vi "Script Cases.vi"(0 "Primitives & Arguments":T1) -> ()   [LabVIEW 2014]
uses:
  Begin/Global Variables.vi
  Begin/Global RefNums.vi
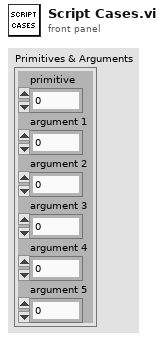
[diagram p1: front panel]
types:
  T1 = cluster{"primitive":i32, "argument 1":dbl, "argument 2":dbl, "argument 3":dbl, "argument 4":dbl, "argument 5":dbl}
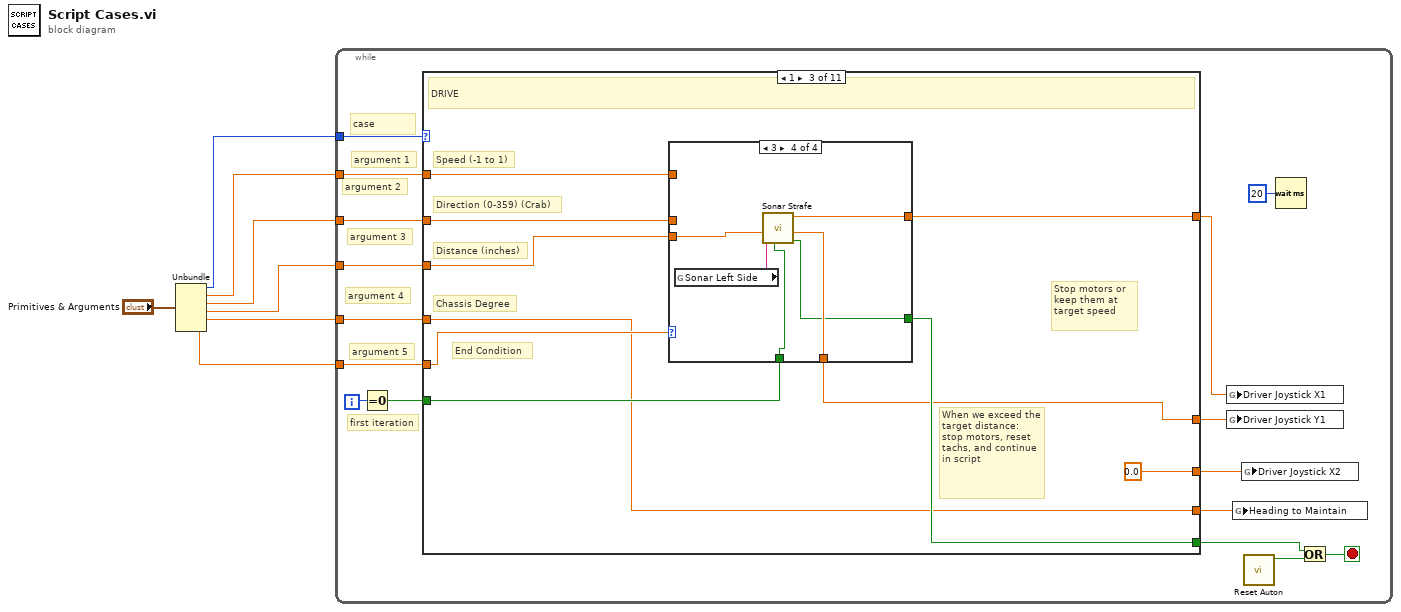
[diagram p0: block diagram]
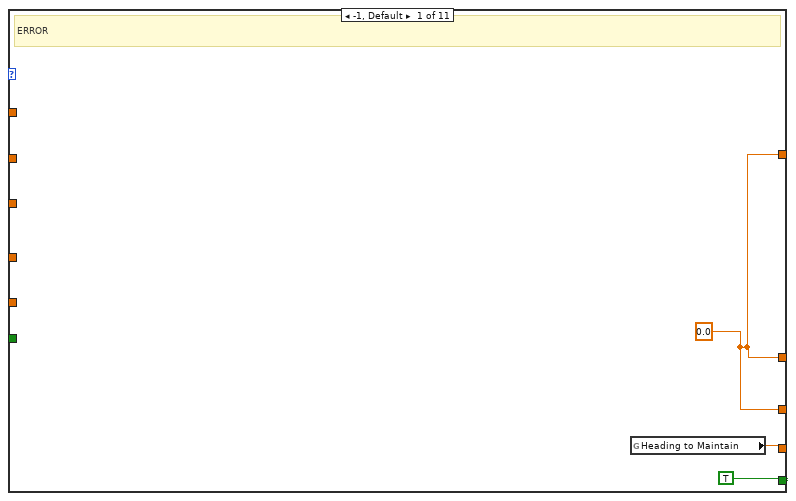
[diagram p2: hidden frame]
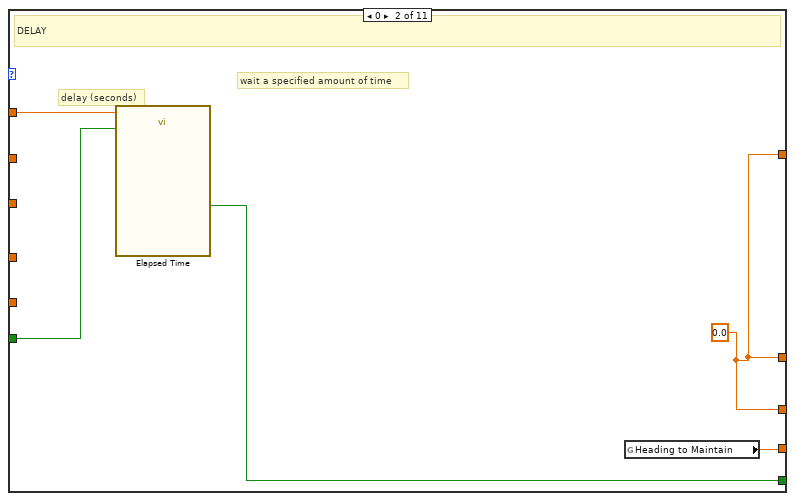
[diagram p3: hidden frame]
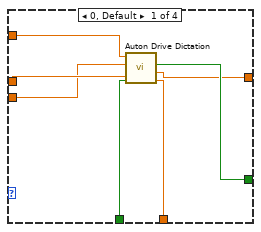
[diagram p4: hidden frame]
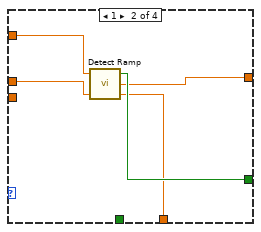
[diagram p5: hidden frame]
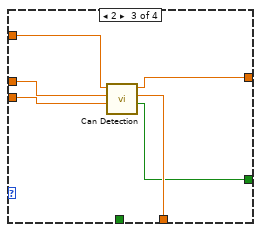
[diagram p6: hidden frame]
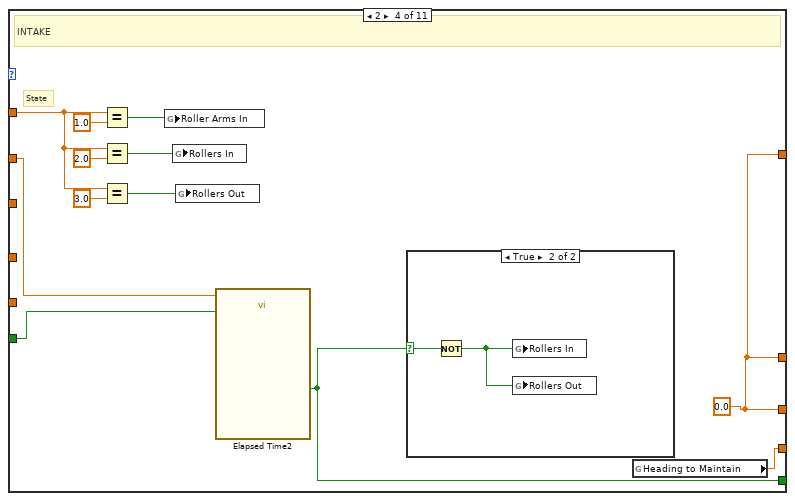
[diagram p7: hidden frame]
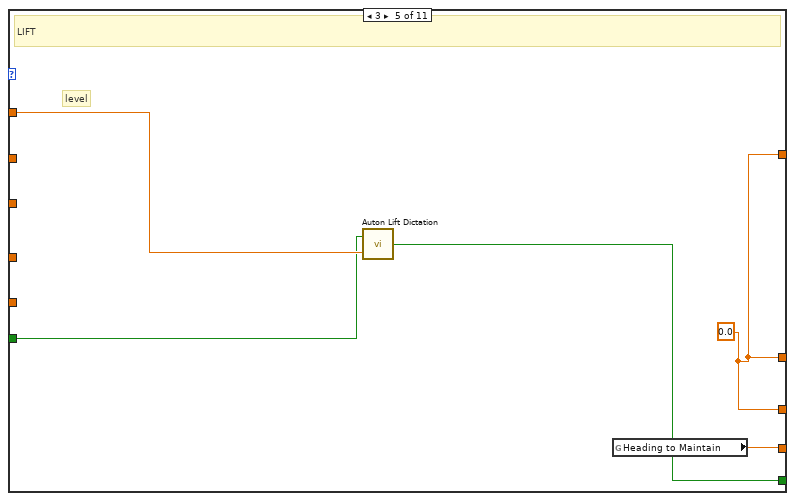
[diagram p9: hidden frame]
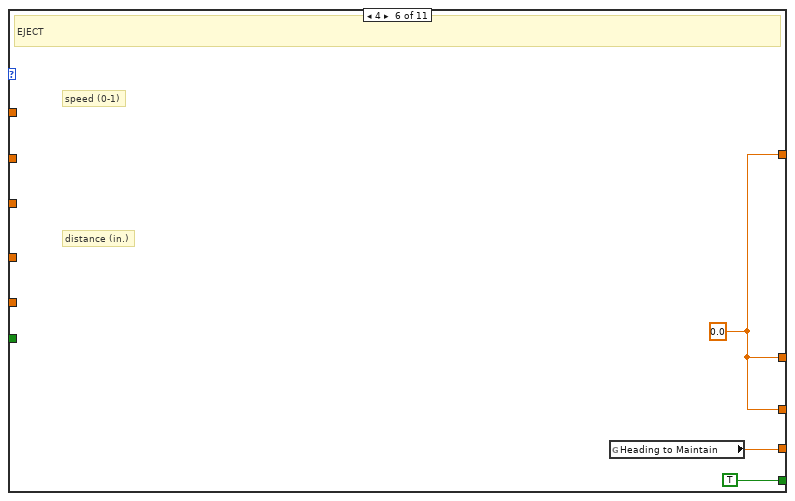
[diagram p10: hidden frame]
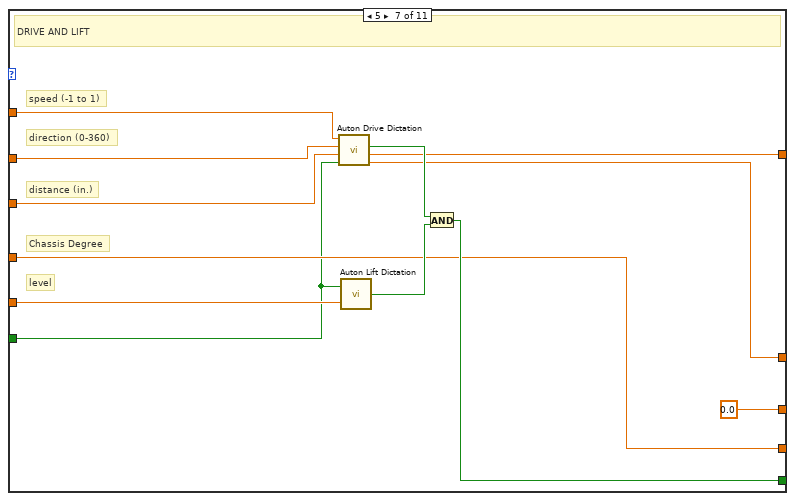
[diagram p11: hidden frame]
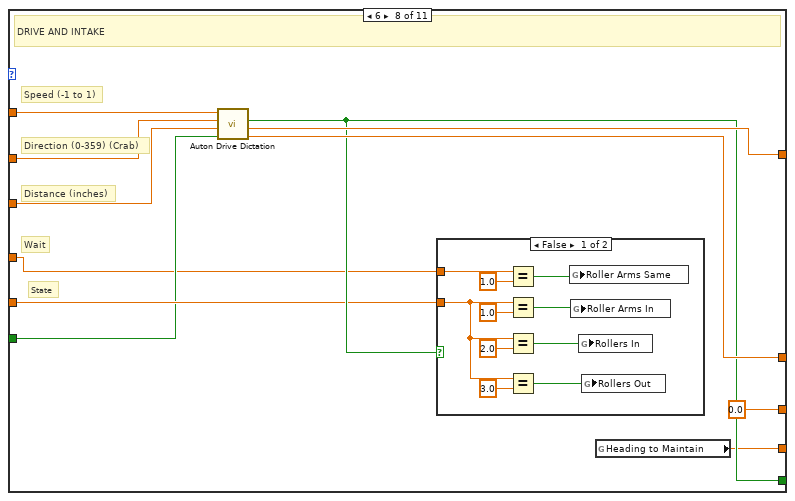
[diagram p12: hidden frame]
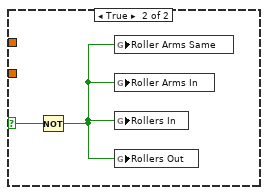
[diagram p13: hidden frame]
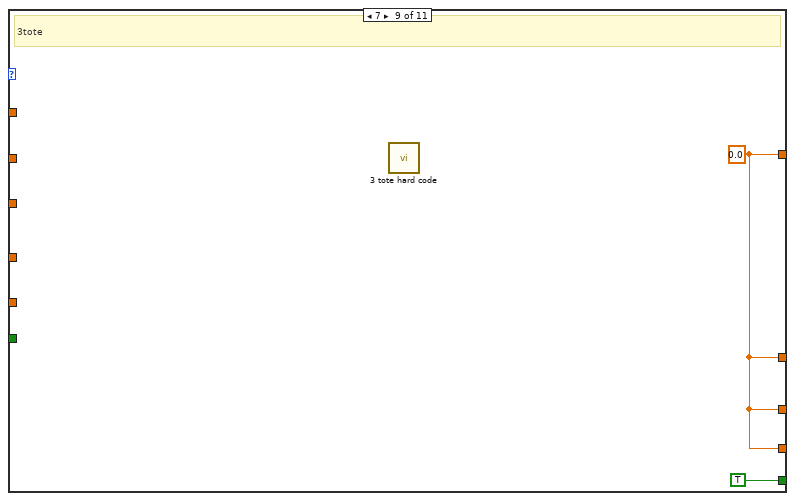
[diagram p14: hidden frame]
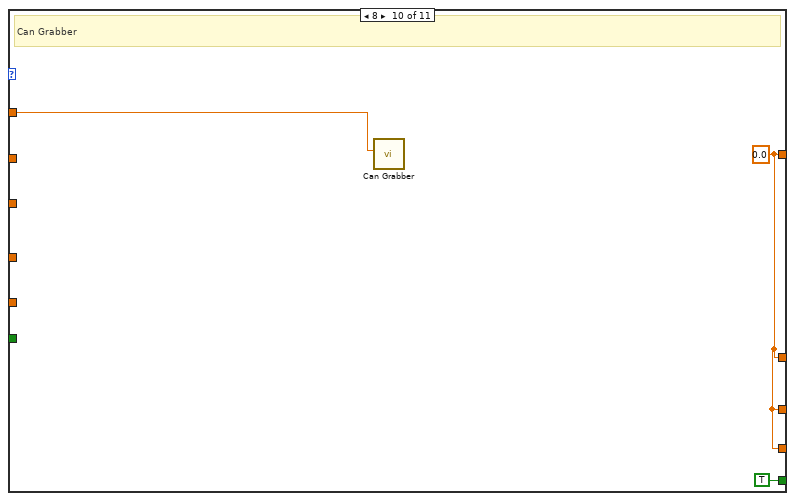
[diagram p15: hidden frame]
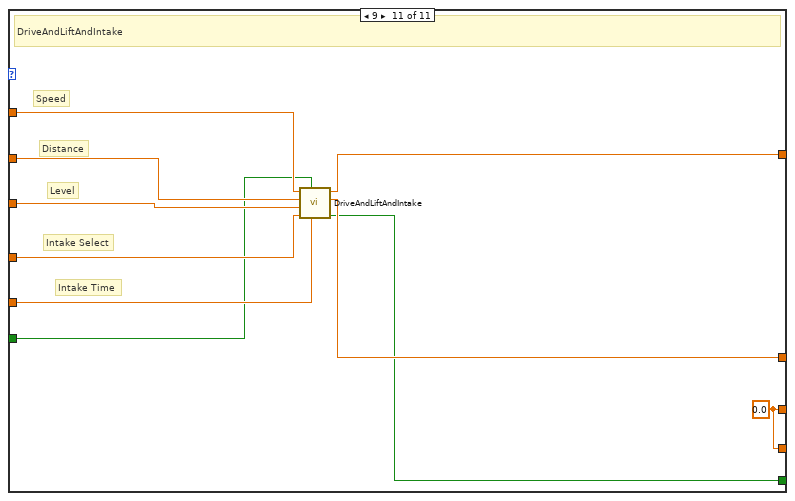
[diagram p16: hidden frame]
diagram:
  n1 = Unbundle("Primitives & Arguments") -> ("primitive"=w6:i32, "argument 1"=w5:dbl, "argument 2"=w4:dbl, "argument 3"=w3:dbl, "argument 4"=w2:dbl, "argument 5"=w1:dbl)
  n2 = while {
    tunnel: w5 -> [w23]
    tunnel: w4 -> [w22]
    tunnel: w3 -> [w21]
    tunnel: w2 -> [w20]
    tunnel: w1 -> [w19]
    tunnel: w6 -> [w18]
    i -> [w17]
    stop <- w9 stop-if-true
    # "first iteration"
    # "case"
    # "argument 5"
    # "argument 4"
    # "argument 3"
    # "argument 2"
    # "argument 1"
    n3 = Equal To 0?(x=w17) -> (x = 0?=w16:bool)
    n4 = case shown="1" w18 {
      tunnel: w23 -> [_ w31 w40 w74 w84 _ w98 w110 _ w125 w137]
      tunnel: w22 -> [_ _ w39 w70 _ _ w97 w109 _ _ w136]
      tunnel: w21 -> [_ _ w38 _ _ _ w96 w108 _ _ w135]
      tunnel: w20 -> [_ _ w34 _ _ _ w89 w101 _ _ w133]
      tunnel: w19 -> [_ _ w35 _ _ _ w95 w103 _ _ w134]
      tunnel: [TRUE w29 w37 w69 w83 TRUE w92 w105 TRUE ("Distance Reached?") TRUE ("Distance Reached?") w130] -> w10
      tunnel: w16 -> [_ w30 w36 w68 w81 _ w88 w102 _ _ w128]
      tunnel: [w25 w28 0.0 ("argument 1") w67 w82 w86 0.0 ("argument 1") 0.0 ("argument 1") w123 w127 w129] -> w15
      tunnel: [w24 w27 w34 w66 w80 w85 w89 w100 w123 w127 w129] -> w14
      tunnel: [w25 w28 w33 w67 w82 w86 w91 w107 w123 w127 w132] -> w12
      tunnel: [w25 w28 w32 w67 w82 w86 w90 w106 w123 w127 w131] -> w11
      frame -1, Default {
        w25 = 0.0 ("argument 1")
        # "ERROR"
        n5 = global read "Global Variables.vi" "Heading to Maintain"() -> (w24:dbl)
      }
      frame 0 {
        w28 = 0.0 ("argument 1")
        # "wait a specified amount of time"
        # "delay (seconds)"
        # "DELAY"
        n6 = call "Elapsed Time"("Time Target (s)"=w31, "Reset"=w30) -> ("Time has Elapsed"=w29:bool)  [unwired: 10 in, 7 out]
        n7 = global read "Global Variables.vi" "Heading to Maintain"() -> (w27:dbl)
      }
      frame 1 {
        # "Chassis Degree"
        # "End Condition"
        # "When we exceed the target distance: stop motors, reset tachs, and continue in script"
        # "Stop motors or keep them at target speed"
        # "Distance (inches)"
        # "Direction (0-359) (Crab)"
        # "Speed (-1 to 1)"
        # "DRIVE"
        n8 = case shown="3" w35 {
          tunnel: w40 -> [w48 w53 w57 _]
          tunnel: w39 -> [w47 w52 w56 _]
          tunnel: w38 -> [w46 _ w55 w65]
          tunnel: [w45 w51 w54 w62] -> w37
          tunnel: w36 -> [w44 _ _ w60]
          tunnel: [w43 w50 w59 w64] -> w33
          tunnel: [w42 w49 w58 w63] -> w32
          frame 0, Default {
            n9 = call "Auton Drive Dictation.vi"("Reset Encoders"=w44, "Distance (inches)"=w46, "Direction (0-359)"=w47, "Speed (-1 to 1)"=w48) -> ("Joy Y"=w42:dbl, "Joy X"=w43:dbl, "Distance Reached?"=w45:bool)  [unwired: 5 in]
          }
          frame 1 {
            n10 = call "Detect Ramp.vi"("Direction"=w52, "Speed"=w53) -> ("JoyY"=w49:dbl, "Joy X"=w50:dbl, "Finished"=w51:bool)  [unwired: 1 in]
          }
          frame 2 {
            n11 = call "Can Detection.vi"("Stop Voltage"=w55, "Direction (0-359)"=w56, "Speed"=w57) -> ("Distance Reached?"=w54:bool, "Joy Y"=w58:dbl, "Joy X"=w59:dbl)  [unwired: 6 in]
          }
          frame 3 {
            n12 = global read "Global RefNums.vi" "Sonar Left Side"() -> (w61:string)
            n13 = call "Sonar Strafe.vi"("reinitialize? (F)"=w60, "Sonar Side"=w61, "Desired Wall Distance"=w65) -> ("Distance Reached?"=w62:bool, "Joy Y"=w63:dbl, "Joy X"=w64:dbl)  [unwired: 6 in]
          }
        }
      }
      frame 2 {
        w67 = 0.0 ("argument 1")
        # "State"
        # "INTAKE"
        n14 = Equal?(x=w74, y=1.0) -> (x = y?=w71:bool)
        n15 = Equal?(x=w74, y=2.0) -> (x = y?=w72:bool)
        n16 = Equal?(x=w74, y=3.0) -> (x = y?=w73:bool)
        n17 = global write "Global Variables.vi" "Roller Arms In"(w71) -> ()
        n18 = global write "Global Variables.vi" "Rollers In"(w72) -> ()
        n19 = global write "Global Variables.vi" "Rollers Out"(w73) -> ()
        n20 = call "Elapsed Time2"("Time Target (s)"=w70, "Reset"=w68) -> ("Time has Elapsed"=w69:bool)  [unwired: 10 in, 7 out]
        n21 = case shown="True" w69 {
          selector: w69 -> [_ w79]
          frame False {
          }
          frame True {
            n22 = Not(x=w79) -> (.not. x?=w78:bool)
            n23 = global write "Global Variables.vi" "Rollers In"(w78) -> ()
            n24 = global write "Global Variables.vi" "Rollers Out"(w78) -> ()
          }
        }
        n25 = global read "Global Variables.vi" "Heading to Maintain"() -> (w66:dbl)
      }
      frame 3 {
        w82 = 0.0 ("argument 1")
        # "level"
        # "LIFT"
        n26 = call "Auton Lift Dictation.vi"("Level"=w84, "First Iteration"=w81) -> ("Lift Sequence Done"=w83:bool)
        n27 = global read "Global Variables.vi" "Heading to Maintain"() -> (w80:dbl)
      }
      frame 4 {
        w86 = 0.0 ("argument 1")
        # "distance (in.)"
        # "speed (0-1)"
        # "EJECT"
        n28 = global read "Global Variables.vi" "Heading to Maintain"() -> (w85:dbl)
      }
      frame 5 {
        # "Chassis Degree"
        # "level"
        # "distance (in.)"
        # "direction (0-360)"
        # "speed (-1 to 1)"
        # "DRIVE AND LIFT"
        n29 = call "Auton Drive Dictation.vi"("Reset Encoders"=w88, "Distance (inches)"=w96, "Direction (0-359)"=w97, "Speed (-1 to 1)"=w98) -> ("Joy Y"=w90:dbl, "Joy X"=w91:dbl, "Distance Reached?"=w94:bool)  [unwired: 5 in]
        n30 = call "Auton Lift Dictation.vi"("Level"=w95, "First Iteration"=w88) -> ("Lift Sequence Done"=w93:bool)
        n31 = And(x=w94, y=w93) -> (x .and. y?=w92:bool)
      }
      frame 6 {
        # "State"
        # "Wait"
        # "Distance (inches)"
        # "Direction (0-359) (Crab)"
        # "Speed (-1 to 1)"
        # "DRIVE AND INTAKE"
        n32 = call "Auton Drive Dictation.vi"("Reset Encoders"=w102, "Distance (inches)"=w108, "Direction (0-359)"=w109, "Speed (-1 to 1)"=w110) -> ("Joy Y"=w106:dbl, "Joy X"=w107:dbl, "Distance Reached?"=w105:bool)  [unwired: 5 in]
        n33 = case shown="False" w105 {
          selector: w105 -> [_ w122]
          tunnel: w103 -> [w114 _]
          tunnel: w101 -> [w111 _]
          frame False {
            n34 = Equal?(x=w111, y=1.0) -> (x = y?=w112:bool)
            n35 = Equal?(x=w114, y=1.0) -> (x = y?=w120:bool)
            n36 = Equal?(x=w114, y=2.0) -> (x = y?=w119:bool)
            n37 = Equal?(x=w114, y=3.0) -> (x = y?=w118:bool)
            n38 = global write "Global Variables.vi" "Roller Arms Same"(w112) -> ()
            n39 = global write "Global Variables.vi" "Roller Arms In"(w120) -> ()
            n40 = global write "Global Variables.vi" "Rollers In"(w119) -> ()
            n41 = global write "Global Variables.vi" "Rollers Out"(w118) -> ()
          }
          frame True {
            n42 = Not(x=w122) -> (.not. x?=w121:bool)
            n43 = global write "Global Variables.vi" "Roller Arms Same"(w121) -> ()
            n44 = global write "Global Variables.vi" "Roller Arms In"(w121) -> ()
            n45 = global write "Global Variables.vi" "Rollers In"(w121) -> ()
            n46 = global write "Global Variables.vi" "Rollers Out"(w121) -> ()
          }
        }
        n47 = global read "Global Variables.vi" "Heading to Maintain"() -> (w100:dbl)
      }
      frame 7 {
        w123 = 0.0 ("Joy X")
        # "3tote"
        n48 = call "3 tote hard code.vi"() -> ()  [unwired: 12 in]
      }
      frame 8 {
        w127 = 0.0 ("Joy X")
        # "Can Grabber"
        n49 = call "Can Grabber.vi"("Grabber State"=w125) -> ()  [unwired: 11 in]
      }
      frame 9 {
        w129 = 0.0 ("Joy X")
        # "Intake Time"
        # "Intake Select"
        # "Level"
        # "Distance"
        # "Speed"
        # "DriveAndLiftAndIntake"
        n50 = call "DriveAndLiftAndIntake.vi"("Intake Time"=w134, "First Iteration"=w128, "Intake Select"=w133, "Level"=w135, "Distance"=w136, "Speed"=w137) -> ("Done?"=w130:bool, "Joy Y"=w131:dbl, "Joy X"=w132:dbl)  [unwired: 3 in]
      }
    }
    n51 = global write "Global Variables.vi" "Driver Joystick X1"(w12) -> ()
    n52 = global write "Global Variables.vi" "Driver Joystick Y1"(w11) -> ()
    n53 = global write "Global Variables.vi" "Heading to Maintain"(w14) -> ()
    n54 = global write "Global Variables.vi" "Driver Joystick X2"(w15) -> ()
    n55 = call "Reset Auton.vi"() -> ("Reset Auton"=w8:bool)  [unwired: 11 in]
    n56 = Wait (ms)(milliseconds to wait=u32 20) -> ()  [unwired: 1 out]
    n57 = Or(x=w10, y=w8) -> (x .or. y?=w9:bool)
  }
